vi "Configure Measurement.vi"(0 "VISA resource name":refnum<visa-resource-name>, 1 "Measurement Time (0.01)":dbl=0.01, 2 "Number of Measurements (1)":i32=1, 5 "Measure Function (0: Frequency)":i32(ring) items=["Frequency", "Burst Carrier Frequency", "Pulse Repetition Frequency", "Fall-time", "Frequency Ratio", "Positive Peak Voltage", "Negative Peak Voltage", "Negative Pulse Width", "Positive Pulse Width", "Positive Duty Cycle", "Negative Duty Cycle", "Phase", "Period", "Rise-time", "Peak-to-Peak Voltage", "Time-Interval", "Power", "Frequency Back-To-Back", "Period Back-To-Back", "TIE"], 7 "Channel  1 (0: A)":i32(ring) items=["A", "B", "C (HF-input option)", "E (Rear panel arming input)", "A prescaled by 2", "Internal Reference", "A with the variable hysteresis mode"], 9 "Channel  2 (0: A)":i32(ring) items=["A", "B", "C (HF-input option)", "E (Rear panel arming input)", "A prescaled by 2", "Internal Reference", "A with the variable hysteresis mode"], 11 "error in (no error)":errorcluster) -> (4 "VISA resource name out":refnum<visa-resource-name>, 15 "error out":errorcluster)   [LabVIEW 2019, in "Pendulum CNT90.lvlib"]
doc: "Configures the type of measurement and selects the input channels and sets the gate time for one measurement."
uses:
  Pendulum CNT90.lvlib
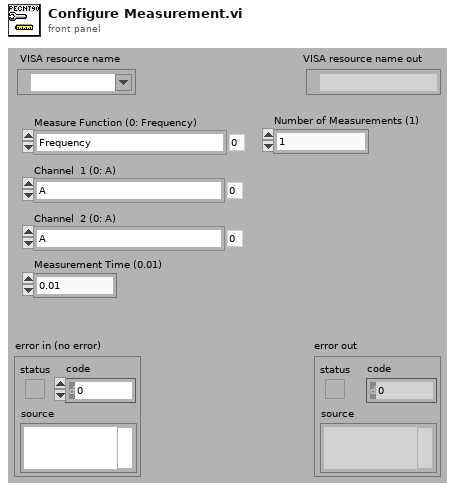
[diagram p1: front panel]
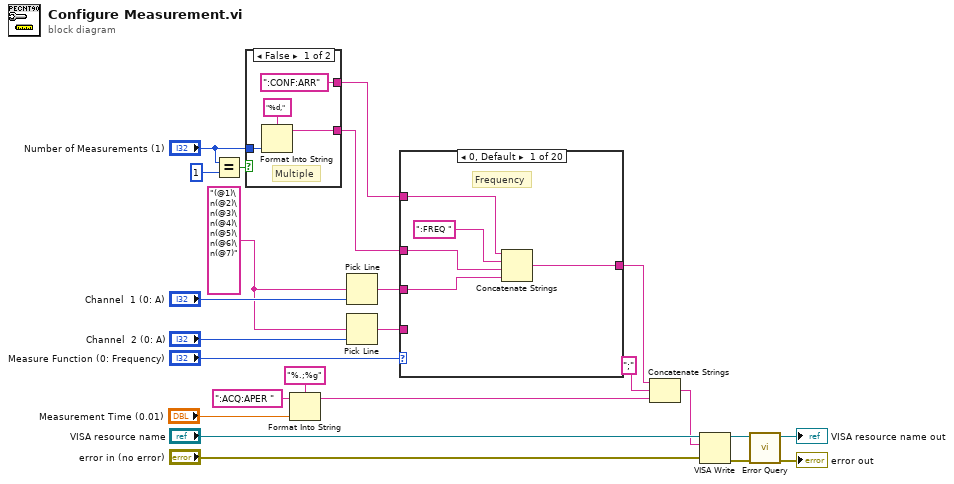
[diagram p0: block diagram]
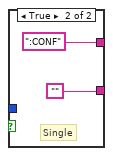
[diagram p2: hidden frame]
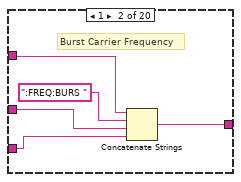
[diagram p3: hidden frame]
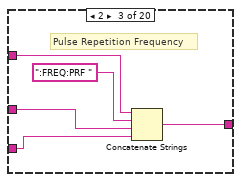
[diagram p4: hidden frame]
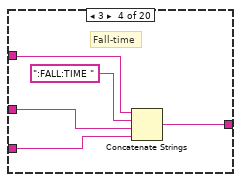
[diagram p5: hidden frame]
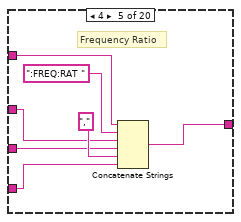
[diagram p6: hidden frame]
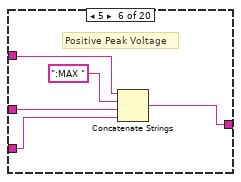
[diagram p7: hidden frame]
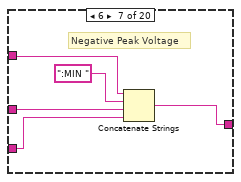
[diagram p8: hidden frame]
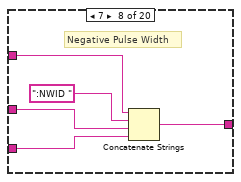
[diagram p9: hidden frame]
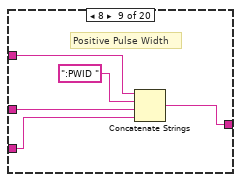
[diagram p10: hidden frame]
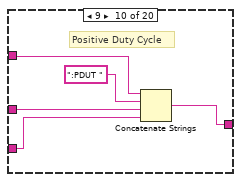
[diagram p11: hidden frame]
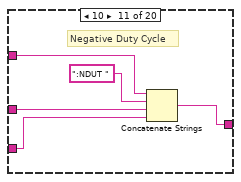
[diagram p12: hidden frame]
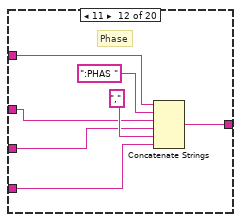
[diagram p13: hidden frame]
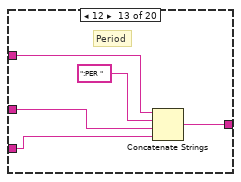
[diagram p14: hidden frame]
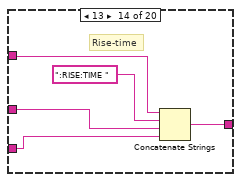
[diagram p15: hidden frame]
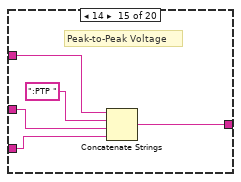
[diagram p16: hidden frame]
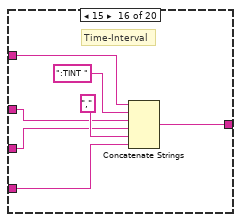
[diagram p17: hidden frame]
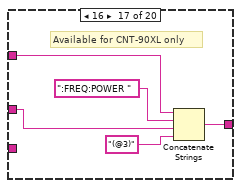
[diagram p18: hidden frame]
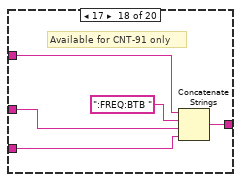
[diagram p19: hidden frame]
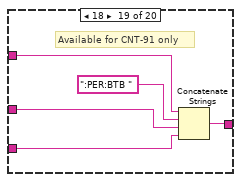
[diagram p20: hidden frame]
diagram:
  w12 = "(@1)\n(@2)\n(@3)\n(@4)\n(@5)\n(@6)\n(@7)"
  n1 = Equal?(x="Number of Measurements (1)", y=1) -> (x = y?=w1:bool)
  n2 = case shown="False" w1 {
    tunnel: [":CONF:ARR" ":CONF"] -> w13
    tunnel: [w26 ""] -> w11
    tunnel: "Number of Measurements (1)" -> [w25 _]
    frame False {
      # "Multiple"
      n3 = Format Into String(format string="%d,", w25) -> (resulting string=w26:string)  [unwired: 2 in, 1 out]
    }
    frame True {
      # "Single"
    }
  }
  n4 = Format Into String(format string="%.;%g", initial string=":ACQ:APER ", "Measurement Time (0.01)") -> (resulting string=w7:string)  [unwired: 1 in, 1 out]
  n5 = Pick Line(multi-line string=w12, line index="Channel  1 (0: A)") -> (output string=w16:string)  [unwired: 1 in]
  n6 = Pick Line(multi-line string=w12, line index="Channel  2 (0: A)") -> (output string=w14:string)  [unwired: 1 in]
  n7 = case shown="0, Default" "Measure Function (0: Frequency)" {
    tunnel: w16 -> [w32 w37 w42 w47 w52 w59 w64 w69 w74 w79 w84 w89 w96 w101 w106 w112 _ w124 w128 w133]
    tunnel: w14 -> [_ _ _ _ w54 _ _ _ _ _ _ w91 _ _ _ w114 _ _ _ _]
    tunnel: w13 -> [w34 w39 w44 w49 w56 w61 w66 w71 w76 w81 w86 w93 w98 w103 w108 w116 w119 w125 w130 w135]
    tunnel: [w33 w38 w43 w48 w55 w60 w65 w70 w75 w80 w85 w92 w97 w102 w107 w115 w118 w122 w127 w132] -> w5
    tunnel: w11 -> [w31 w36 w41 w46 w51 w58 w63 w68 w73 w78 w83 w88 w95 w100 w105 w111 w117 w123 w129 w134]
    frame 0, Default {
      # "Frequency"
      n8 = Concatenate Strings(w34, ":FREQ ", w31, w32) -> (w33:string)
    }
    frame 1 {
      # "Burst Carrier Frequency"
      n9 = Concatenate Strings(w39, ":FREQ:BURS ", w36, w37) -> (w38:string)
    }
    frame 2 {
      # "Pulse Repetition Frequency"
      n10 = Concatenate Strings(w44, ":FREQ:PRF ", w41, w42) -> (w43:string)
    }
    frame 3 {
      # "Fall-time"
      n11 = Concatenate Strings(w49, ":FALL:TIME ", w46, w47) -> (w48:string)
    }
    frame 4 {
      # "Frequency Ratio"
      n12 = Concatenate Strings(w56, ":FREQ:RAT ", w51, w52, "," ("string"), w54) -> (w55:string)
    }
    frame 5 {
      # "Positive Peak Voltage"
      n13 = Concatenate Strings(w61, ":MAX ", w58, w59) -> (w60:string)
    }
    frame 6 {
      # "Negative Peak Voltage"
      n14 = Concatenate Strings(w66, ":MIN ", w63, w64) -> (w65:string)
    }
    frame 7 {
      # "Negative Pulse Width"
      n15 = Concatenate Strings(w71, ":NWID ", w68, w69) -> (w70:string)
    }
    frame 8 {
      # "Positive Pulse Width"
      n16 = Concatenate Strings(w76, ":PWID ", w73, w74) -> (w75:string)
    }
    frame 9 {
      # "Positive Duty Cycle"
      n17 = Concatenate Strings(w81, ":PDUT ", w78, w79) -> (w80:string)
    }
    frame 10 {
      # "Negative Duty Cycle"
      n18 = Concatenate Strings(w86, ":NDUT ", w83, w84) -> (w85:string)
    }
    frame 11 {
      # "Phase"
      n19 = Concatenate Strings(w93, ":PHAS ", w88, w89, "," ("string"), w91) -> (w92:string)
    }
    frame 12 {
      # "Period"
      n20 = Concatenate Strings(w98, ":PER ", w95, w96) -> (w97:string)
    }
    frame 13 {
      # "Rise-time"
      n21 = Concatenate Strings(w103, ":RISE:TIME ", w100, w101) -> (w102:string)
    }
    frame 14 {
      # "Peak-to-Peak Voltage"
      n22 = Concatenate Strings(w108, ":PTP ", w105, w106) -> (w107:string)
    }
    frame 15 {
      # "Time-Interval"
      n23 = Concatenate Strings(w116, ":TINT ", w111, w112, "," ("string"), w114) -> (w115:string)
    }
    frame 16 {
      # "Available for CNT-90XL only"
      n24 = Concatenate Strings(w119, ":FREQ:POWER ", w117, "(@3)") -> (w118:string)
    }
    frame 17 {
      # "Available for CNT-91 only"
      n25 = Concatenate Strings(w125, ":FREQ:BTB ", w123, w124) -> (w122:string)
    }
    frame 18 {
      # "Available for CNT-91 only"
      n26 = Concatenate Strings(w130, ":PER:BTB ", w129, w128) -> (w127:string)
    }
    frame 19 {
      # "Available for CNT-91 only"
      n27 = Concatenate Strings(w135, ":TIE ", w134, w133) -> (w132:string)
    }
  }
  n28 = Concatenate Strings(w5, ";", w7) -> (w4:string)
  n29 = VISA Write(VISA resource name="VISA resource name", write buffer=w4, error in (no error)="error in (no error)") -> (VISA resource name out=w22:refnum<visa-resource-name>, error out=w19:errorcluster)  [unwired: 1 out]
  n30 = call "Error Query.vi"("error in (no error)"=w19, "VISA resource name"=w22) -> ("error out"=→"error out":errorcluster, "VISA resource name out"=→"VISA resource name out":refnum<visa-resource-name>)  [unwired: 6 in, 2 out]
